vi "uTTA_GetPWUVLO.vi"(8 "error in":errorcluster, 11 "VISA Refnum in":refnum<visa-resource-name>) -> (0 "error out":errorcluster, 1 "Powerstage Undervoltage":bool, 2 "Received":string, 3 "VISA Refnum out":refnum<visa-resource-name>)   [LabVIEW 2021]
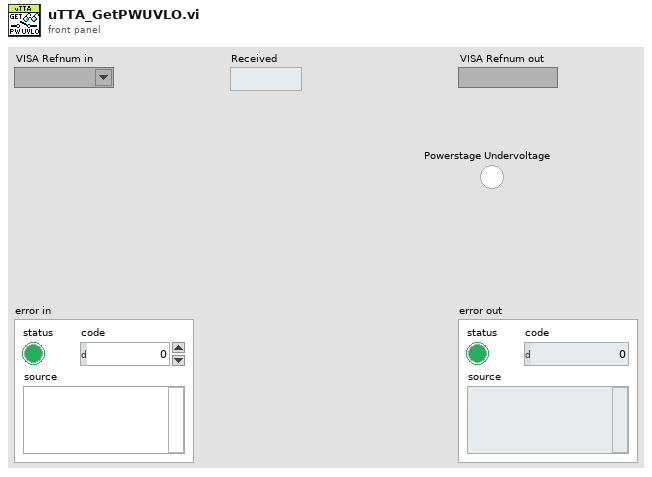
[diagram p1: front panel]
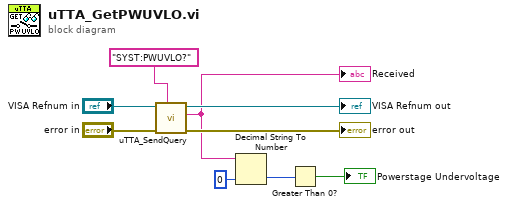
[diagram p0: block diagram]
diagram:
  n1 = call "uTTA_SendQuery.vi"("Send String"="SYST:PWUVLO?" ("format string"), "error in (no error)"="error in", "VISA Refnum in"="VISA Refnum in") -> ("error out"=→"error out":errorcluster, "Received"=w6:string, "VISA Refnum out"=→"VISA Refnum out":refnum<visa-resource-name>)  [unwired: 6 in]
  "Received" <- w6
  n2 = Decimal String To Number(string=w6, default (0L)=0 ("default (0 I32)")) -> (number=w4:i32)  [unwired: 1 in, 1 out]
  n3 = Greater Than 0?(x=w4) -> (x > 0?=→"Powerstage Undervoltage":bool)
